vi "Cross Board Game With Shield.vi"(6 "Max Shield?":bool, 9 "y":dbl, 11 "x":dbl) -> (1 "y out":dbl, 3 "x out":dbl, 4 "Crossed?":bool)   [LabVIEW 2021, in "Board Game.lvclass"]
uses:
  Board Game.lvclass
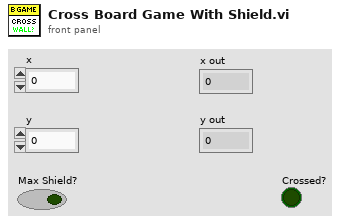
[diagram p1: front panel]
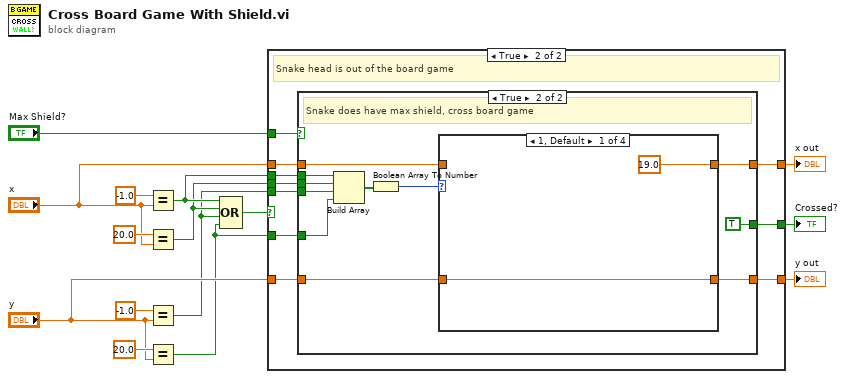
[diagram p0: block diagram]
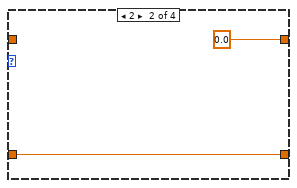
[diagram p4: hidden frame]
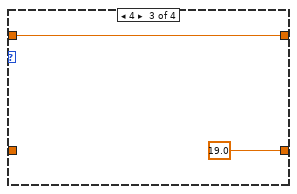
[diagram p5: hidden frame]
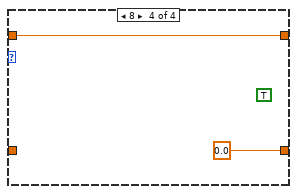
[diagram p6: hidden frame]
diagram:
  n1 = Equal?(x=-1.0, y="x") -> (x = y?=w6:bool)
  n2 = Equal?(x=20.0, y="x") -> (x = y?=w5:bool)
  n3 = Equal?(x=-1.0, y="y") -> (x = y?=w4:bool)
  n4 = Equal?(x=20.0, y="y") -> (x = y?=w3:bool)
  n5 = Compound Arithmetic op=OR(w6, w5, w4, w3) -> (w11:bool)
  n6 = case shown="True" w11 {
    tunnel: "x" -> [w16 w22]
    tunnel: "y" -> [w17 w23]
    tunnel: [w17 w20] -> w7
    tunnel: [w16 w21] -> w8
    tunnel: w6 -> [_ w27]
    tunnel: w5 -> [_ w26]
    tunnel: w4 -> [_ w25]
    tunnel: w3 -> [_ w24]
    tunnel: "Max Shield?" -> [_ w19]
    tunnel: [_ w18] -> w1
    frame False {
      # "Snake head is not out of the board game"
    }
    frame True {
      # "Snake head is out of the board game"
      n7 = case shown="True" w19 {
        tunnel: w27 -> [_ w40]
        tunnel: w26 -> [_ w39]
        tunnel: w25 -> [_ w38]
        tunnel: w24 -> [_ w37]
        tunnel: w23 -> [w28 w34]
        tunnel: w22 -> [w29 w33]
        tunnel: [w29 w32] -> w21
        tunnel: [w28 w31] -> w20
        tunnel: [_ TRUE] -> w18
        frame False {
          # "Snake does not have max shield"
        }
        frame True {
          # "Snake does have max shield, cross board game"
          n8 = Build Array(w40, w39, w38, w37) -> (w36:bool[])
          n9 = Boolean Array To Number(Boolean array=w36) -> (number=w35:u32)
          n10 = case shown="1, Default" w35 {
            tunnel: w34 -> [w42 w44 _ _]
            tunnel: w33 -> [_ _ w45 w48]
            tunnel: [19.0 ("x") 0.0 ("x") w45 w48] -> w32
            tunnel: [w42 w44 19.0 ("x") 0.0 ("x")] -> w31
            frame 1, Default {
            }
            frame 2 {
            }
            frame 4 {
            }
            frame 8 {
              (unwired) TRUE
            }
          }
        }
      }
    }
  }
  "x out" <- w8
  "y out" <- w7
  "Crossed?" <- w1
